vi "GetConfigChain.vi"(8 "error in (no error)":errorcluster, 11 "reference in":refnum<class "JTAG_Cyclone.lvclass">) -> (0 "error out":errorcluster, 2 "Config out":string[](array[string]), 3 "reference out":refnum<class "JTAG_Cyclone.lvclass">)   [LabVIEW 2022 SP3, in "JTAG_Cyclone.lvlib" / "JTAG_Cyclone.lvclass"]
uses:
  JTAG_Cyclone.lvclass
  Components/JTAG_Base.lvlibp/JTAG_Base.lvclass
  Components/ViPER.lvlibp/ViPER.lvclass
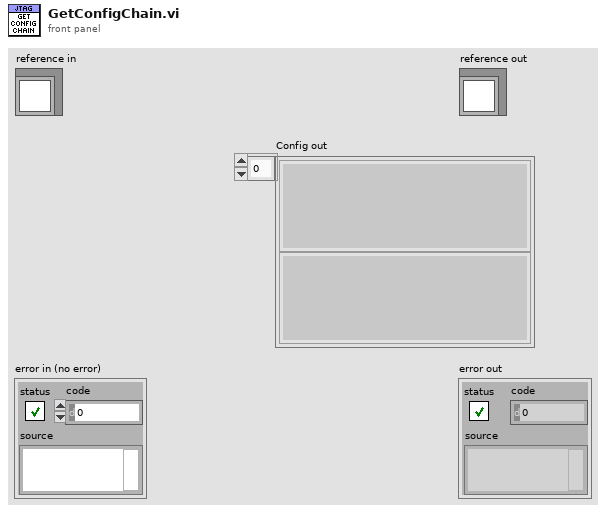
[diagram p1: front panel]
types:
  T1 = typedef "JTAG_Cyclone.lvlib/JTAG_Cyclone.lvclass/ObjectAttributes.ctl" = cluster{"Config":T2, "Success":bool, "Msg":string, "active image":string}
  T2 = typedef "JTAG_Cyclone.lvlib/JTAG_Cyclone.lvclass/Config.ctl" = cluster{"Cyclone_API_Path":path, "Cyclone_Name":string}
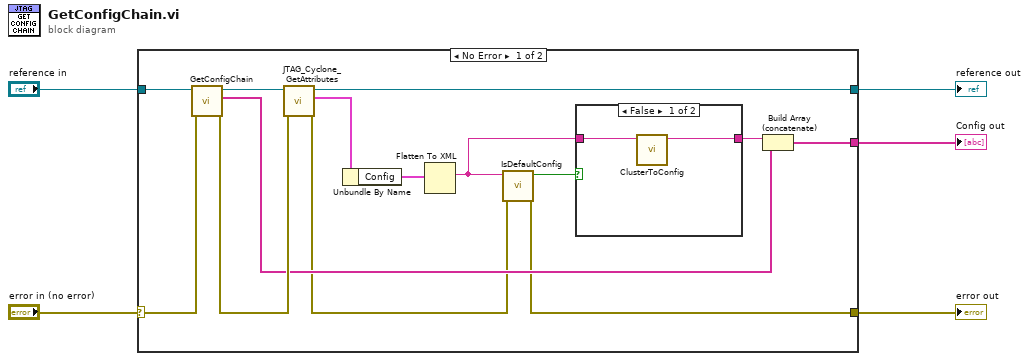
[diagram p0: block diagram]
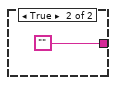
[diagram p2: hidden frame]
diagram:
  n1 = case shown="No Error" "error in (no error)" {
    selector: "error in (no error)" -> [w15 w24]
    tunnel: [w6 w24] -> w4
    tunnel: [w13 w23] -> w2
    tunnel: "reference in" -> [w17 w23]
    tunnel: [w10 _] -> w1
    frame No Error {
      n2 = call-parent "GetConfigChain.vi"("error in (no error)"=w15, "reference in"=w17) -> ("error out"=w14:errorcluster, "Config out"=w11:string[], "reference out"=w16:refnum<class "JTAG_Cyclone.lvclass">)  [unwired: 7 in]
      n3 = call "JTAG_Cyclone_GetAttributes.vi"("error in (no error)"=w14, "reference in"=w16) -> ("error out"=w7:errorcluster, "Data"=w19:T1, "reference out"=w13:refnum<class "JTAG_Cyclone.lvclass">)  [unwired: 6 in, 1 out]
      n4 = Unbundle By Name(w19) -> ("Config"=w18:T2)
      n5 = Flatten To XML(6:w18) -> (2:w9:string)
      n6 = call "IsDefaultConfig.vi"("error in (no error)"=w7, "Config XML"=w9) -> ("error out"=w6:errorcluster, "Is Default"=w8:bool)  [unwired: 8 in]
      n7 = case shown="False" w8 {
        tunnel: w9 -> [w21 _]
        tunnel: [w20 ""] -> w12
        frame False {
          n8 = call "ClusterToConfig.vi"("Cluster XML"=w21) -> ("Config XML"=w20:string)  [unwired: 10 in]
        }
        frame True {
        }
      }
      n9 = Build Array (concatenate)(w12, w11) -> (w10:string[])
    }
    frame Error {
    }
  }
  "error out" <- w4
  "reference out" <- w2
  "Config out" <- w1
